vi "Generate Test Data.vi"(11 "Vaisala Data in":refnum<class "Vaisala Data.lvclass">) -> (3 "Vaisala Data out":refnum<class "Vaisala Data.lvclass">)   [LabVIEW 2014, in "Vaisala Library.lvlib" / "Vaisala Data.lvclass"]
uses:
  Vaisala Data.lvclass
  Vaisala Data.lvclass/Vaisala Data.ctl
  reusable/Data/Data.lvclass
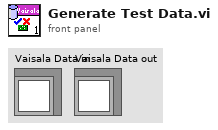
[diagram p1: front panel]
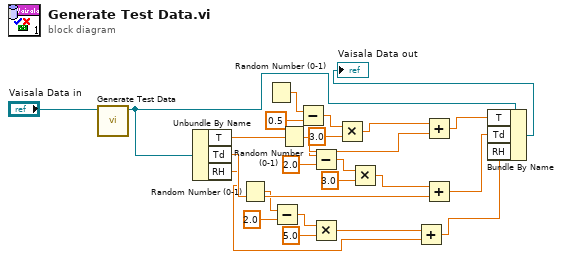
[diagram p0: block diagram]
diagram:
  n1 = call-parent "Generate Test Data.vi"("Data in"="Vaisala Data in") -> ("Data out"=w5:refnum<class "Vaisala Data.lvclass">)  [unwired: 10 in]
  n2 = Unbundle By Name(w5) -> ("T"=w18:dbl, "Td"=w17:dbl, "RH"=w6:dbl)
  n3 = Random Number (0-1)() -> (number: 0 to 1=w10:dbl)
  n4 = Random Number (0-1)() -> (number: 0 to 1=w23:dbl)
  n5 = Subtract(x=w10, y=2.0) -> (x-y=w8:dbl)
  n6 = Random Number (0-1)() -> (number: 0 to 1=w14:dbl)
  n7 = Subtract(x=w23, y=0.5) -> (x-y=w21:dbl)
  n8 = Subtract(x=w14, y=2.0) -> (x-y=w16:dbl)
  n9 = Multiply(x=w8, y=5.0) -> (x*y=w7:dbl)
  n10 = Multiply(x=w21, y=3.0) -> (x*y=w19:dbl)
  n11 = Multiply(x=w16, y=3.0) -> (x*y=w12:dbl)
  n12 = Add(x=w7, y=w6) -> (x+y=w2:dbl)
  n13 = Add(x=w19, y=w18) -> (x+y=w4:dbl)
  n14 = Add(x=w12, y=w17) -> (x+y=w3:dbl)
  n15 = Bundle By Name(cluster=w5, "T"=w4, "Td"=w3, "RH"=w2) -> (→"Vaisala Data out":refnum<class "Vaisala Data.lvclass">)
